vi "Main.vi"() -> ()   [LabVIEW 2020]
doc: "Ce VI modèle est conçu pour le modèle de conception Gestionnaire de messages dans une file d'attente.\n\nLa boucle de gestion d'événements génère des messages en fonction des actions sur l'interface utilisateur.\n\nLa boucle de gestion de messages traite les messages générés par la boucle de gestion d'événements ou par d'autres messages. Les messages sont des valeurs chaîne ; il est donc facile d'ajouter de nouveaux messages à la structure condition Conditions de messages de la boucle de gestion de messages Chaque cluster Message peut en outre fournir une valeur optionnelle pour Données de message, un variant qui peut être converti aux données requises pour un message spécifique."
uses:
  controls/Ctrl_Display.ctl
  controls/Ctrl_RefPad.ctl
  <vilib>/Utility/error.llb/Error Cluster From Error Code.vi
  support/Message Queue/Enqueue Message (Single).vi
  <vilib>/ErrorRing/Error Ring.xnode
  support/Message Queue/Message Queue.lvlib
  support/User Event - Stop/User Event - Stop.lvlib
panel:
  out "sortie d'erreur 2":errorcluster caption="sortie d'erreur"
  in  "Btn_Error_etat":bool caption="Error state"
  in  "Btn_Error":bool caption="Error"
  out "sortie d'erreur":errorcluster
  out "Display":T1
  in  "Pad":T2
  in  "Btn_Stop":bool
  # "Calculatrice"
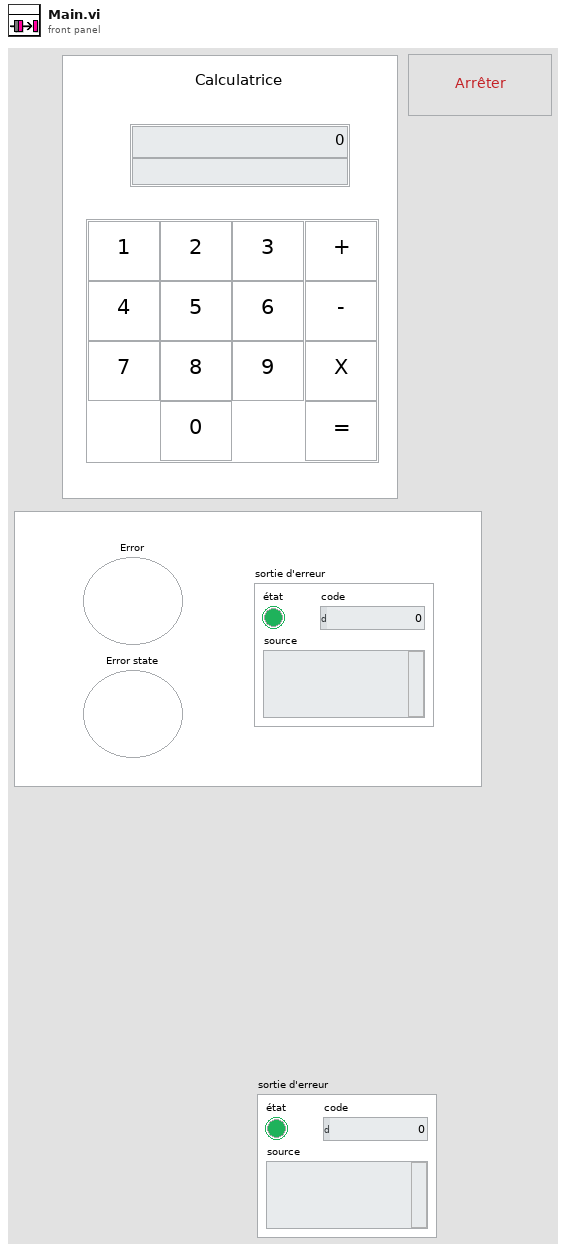
[diagram p1: front panel]
types:
  T1 = typedef "Ctrl_Display.ctl" = cluster{"Num":dbl, "Char":string}
  T2 = cluster{"Btn_1":bool, "Btn_2":bool, "Btn_3":bool, "Btn_4":bool, "Btn_5":bool, "Btn_6":bool, "Btn_7":bool, "Btn_8":bool, "Btn_9":bool, "Btn_0":bool, "Btn_+":bool, "Btn_-":bool, "Btn_X":bool, "Btn_=":bool}
  T3 = cluster{"état":bool, "code":i32, "source":string}
  T4 = typedef "Message Queue.lvlib/All Message Queues.ctl" = cluster{"Conductor":refnum<queue>, "IU":refnum<queue>}
  T5 = typedef "Ctrl_RefPad.ctl" = cluster{"BTN_Ref":refnum<vi>, "CharPad":string}
  T6 = typedef "UI Data.ctl" = cluster{"Data":cluster{"memory":string, "Display":T1}, "Ref":T7}
  T7 = typedef "Ctrl_Ref.ctl" = cluster{"Fifo":T4, "Event":cluster{"Stop":refnum<user-event>}}
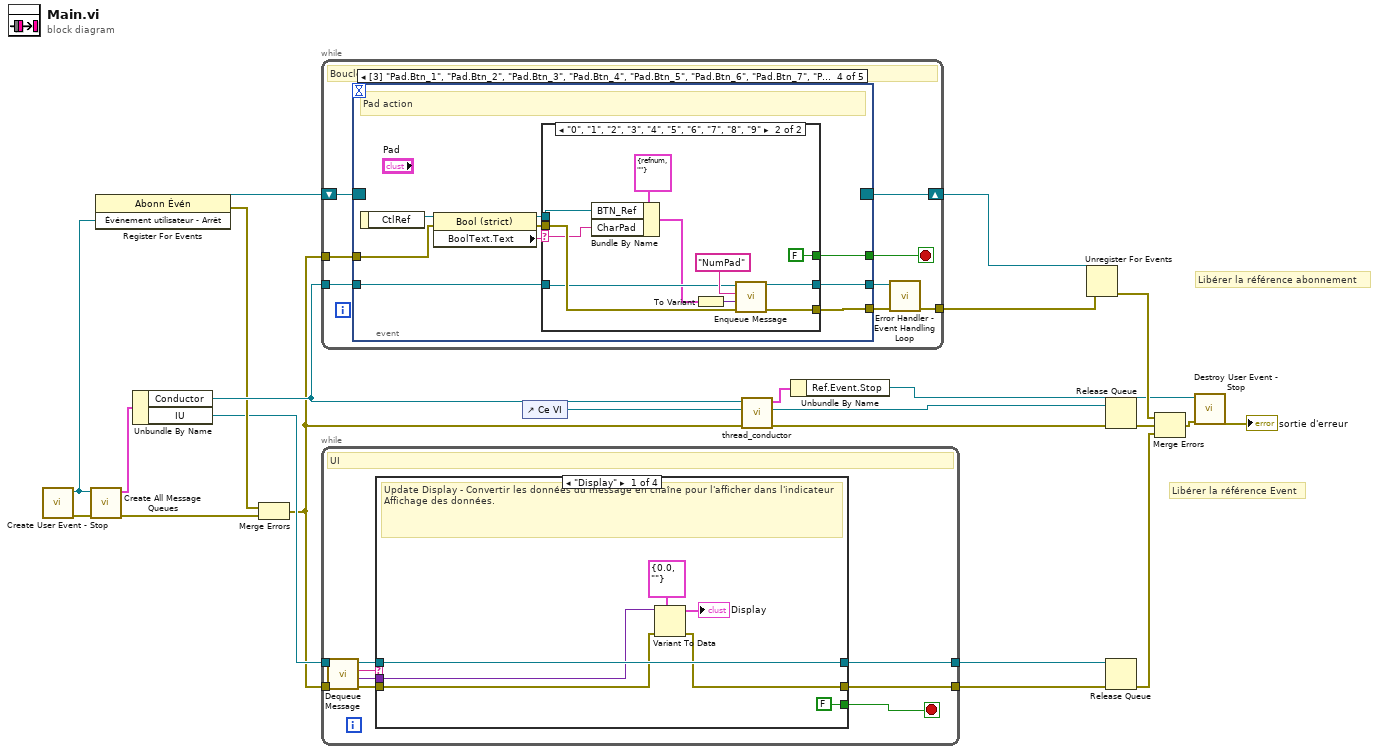
[diagram p0: block diagram]
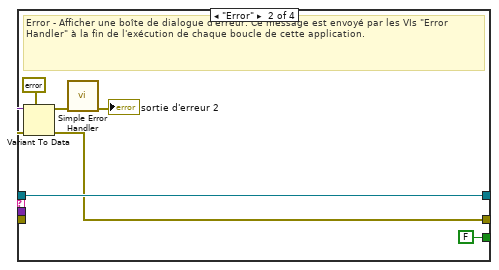
[diagram p2: hidden frame]
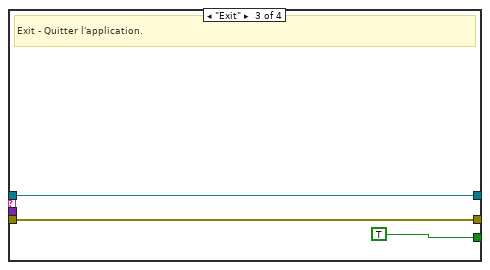
[diagram p3: hidden frame]
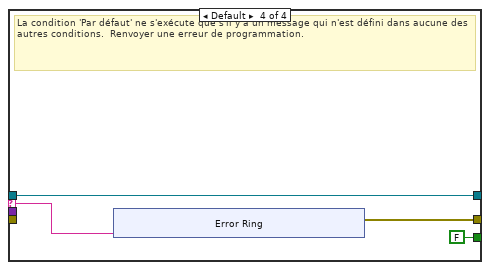
[diagram p4: hidden frame]
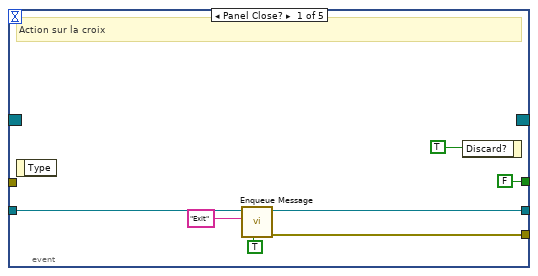
[diagram p5: hidden frame]
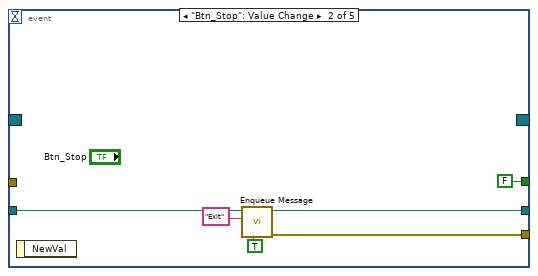
[diagram p6: hidden frame]
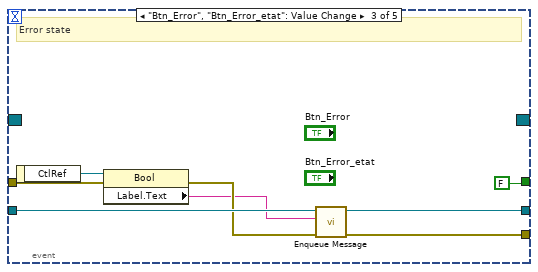
[diagram p7: hidden frame]
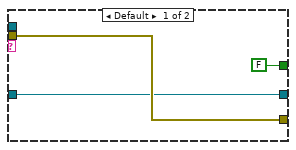
[diagram p8: hidden frame]
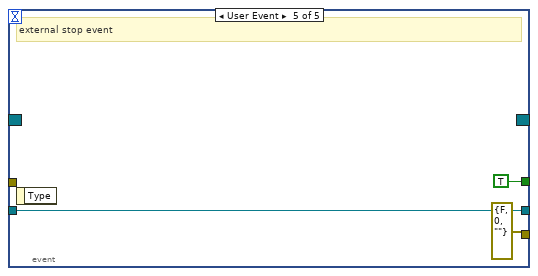
[diagram p9: hidden frame]
diagram:
  # "Libérer la référence abonnement"
  # "Libérer la référence Event"
  n1 = call "Create User Event - Stop.vi"() -> ("error out"=w20:T3, "Événement utilisateur - Arrêt"=w13:refnum<user-event>)  [unwired: 10 in]
  n2 = call "Create All Message Queues.vi"("error in (no error)"=w20, "Stop Event"=w13) -> ("error out"=w23:T3, "Fifo"=w22:T4)  [unwired: 8 in]
  n3 = register-events(w13) -> (reference out=w15:refnum<event-registration>, error out=w14:errorcluster)  [unwired: 2 in]
  n4 = Unbundle By Name(w22) -> ("Conductor"=w21:refnum<queue>, "IU"=w9:refnum<queue>)
  n5 = Merge Errors(w14, w23) -> (w8:errorcluster)
  n6 = while {
    tunnel: w21 -> [w31]
    shift-right: [w29] -> w17
    shift-left: w15 -> [w30]
    tunnel: [w25] -> w16
    tunnel: w8 -> [w24]
    stop <- w27 stop-if-true
    # "Boucle de gestion d'événements"
    n7 = event shown="[3] \"Pad.Btn_1\", \"Pad.Btn_2\", \"Pad.Btn_3\", \"Pad.Btn_4\", \"Pad.Btn_5\", \"Pad.Btn_6\", \"Pad.Btn_7\", \"Pad.Btn_8\", \"Pad.Btn_9\", \"Pad.Btn_0\", \"Pad.Btn_+\": Valeur changée" {
      selector: w30 -> [_ _ _ _ _]
      dyn-events: [_ _ _ _ _] -> w29
      timeout: _ -> [_ _ _ _ _]
      tunnel: [FALSE ("Discard?") FALSE ("Discard?") FALSE w54 TRUE ("Discard?")] -> w27
      tunnel: w31 -> [w37 w44 w50 w56 w78]
      tunnel: [w36 w43 w45 w57 T3 {"état"=FALSE, "code"=0, "source"=""} ("error out")] -> w28
      tunnel: [w35 w42 w49 w55 w78] -> w26
      tunnel: w24 -> [_ _ w51 w60 _]
      event Panel Close? {
        # "Action sur la croix"
        n8 = event-data() -> ()  [unwired: 1 in, 1 out]
        n9 = call-poly "Enqueue Message.vi"("Message prioritaire ? (F)"=TRUE ("Priority Message? (F)"), "Message"="Exit", "File d'attente de messages"=w37) -> ("error out"=w36:T3, "File d'attente de message dup."=w35:refnum<queue>)  [unwired: 7 in]
        n10 = event-data ("Event Filter Node")("Discard?"=TRUE) -> ()  [unwired: 1 in, 1 out]
      }
      event "Btn_Stop": Value Change {
        n11 = event-data() -> ()  [unwired: 1 in, 1 out]
        n12 = call-poly "Enqueue Message.vi"("Message prioritaire ? (F)"=TRUE ("Priority Message? (F)"), "Message"="Exit", "File d'attente de messages"=w44) -> ("error out"=w43:T3, "File d'attente de message dup."=w42:refnum<queue>)  [unwired: 7 in]
      }
      event "Btn_Error", "Btn_Error_etat": Value Change {
        # "Error state"
        n13 = event-data() -> ("CtlRef"=w52:refnum<vi>)  [unwired: 1 in]
        n14 = property class="Bool"(reference=w52, error in=w51) -> (error out=w48:errorcluster, "Label.Text"=w47:string)  [unwired: 1 out]
        n15 = call-poly "Enqueue Message.vi"("error in (no error)"=w48, "Message"=w47, "File d'attente de messages"=w50) -> ("error out"=w45:T3, "File d'attente de message dup."=w49:refnum<queue>)  [unwired: 7 in]
      }
      event "Pad.Btn_1", "Pad.Btn_2", "Pad.Btn_3", "Pad.Btn_4", "Pad.Btn_5", "Pad.Btn_6", "Pad.Btn_7", "Pad.Btn_8", "Pad.Btn_9", "Pad.Btn_0", "Pad.Btn_+": Value Change {
        # "Pad action"
        n16 = event-data() -> ("CtlRef"=w61:refnum<vi>)  [unwired: 1 in]
        n17 = property class="Bool (strict)"(reference=w61, error in=w60) -> (reference out=w53:refnum<vi>, error out=w58:errorcluster, "BoolText.Text"=w59:string)
        n18 = case shown="\"0\", \"1\", \"2\", \"3\", \"4\", \"5\", \"6\", \"7\", \"8\", \"9\"" w59 {
          selector: w59 -> [_ w67]
          tunnel: w58 -> [w64 w74]
          tunnel: [w64 w73] -> w57
          tunnel: w56 -> [w63 w71]
          tunnel: [w63 w70] -> w55
          tunnel: [FALSE FALSE] -> w54
          tunnel: w53 -> [_ w68]
          frame Default {
          }
          frame "0", "1", "2", "3", "4", "5", "6", "7", "8", "9" {
            n19 = Bundle By Name(cluster=T5 {"BTN_Ref"=refnum, "CharPad"=""}, "BTN_Ref"=w68, "CharPad"=w67) -> (w66:T5)
            n20 = To Variant(anything=w66) -> (Variant=w72:variant)
            n21 = call-poly "Enqueue Message.vi"("error in (no error)"=w74, "Données de message"=w72, "Message"="NumPad", "File d'attente de messages"=w71) -> ("error out"=w73:T3, "File d'attente de message dup."=w70:refnum<queue>)  [unwired: 6 in]
          }
        }
      }
      event User Event {
        # "external stop event"
        n22 = event-data() -> ()  [unwired: 1 in, 1 out]
      }
    }
    n23 = call "Error Handler - Event Handling Loop.vi"("error in (no error)"=w28, "File d'attente de messages"=w26) -> ("erreur en entrée dup."=w25:T3)  [unwired: 8 in, 1 out]
  }
  n24 = while {
    tunnel: w9 -> [w85]
    tunnel: w8 -> [w86]
    tunnel: [w79] -> w6
    tunnel: [w80] -> w7
    stop <- w87 stop-if-true
    # "UI"
    n25 = call "Dequeue Message.vi"("error in (no error)"=w86, "File d'attente de messages"=w85) -> ("error out"=w84:T3, "Données de message"=w82:variant, "Message"=w83:string, "File d'attente de message dup."=w81:refnum<queue>)  [unwired: 6 in]
    n26 = case "Conditions des messages" shown="\"Display\"" w83 {
      selector: w83 -> [_ _ _ w108]
      tunnel: w81 -> [w93 w96 w104 w106]
      tunnel: w84 -> [w92 w102 w103 _]
      tunnel: [w91 w95 w103 w109] -> w79
      tunnel: [FALSE FALSE TRUE FALSE] -> w87
      tunnel: w82 -> [w90 w101 _ _]
      tunnel: [w93 w96 w104 w106] -> w80
      frame "Display" {
        # "Update Display - Convertir les données du message en chaîne pour l'afficher dans l'indicateur Affichage des données."
        n27 = Variant To Data(error in=w92, type=T1 {"Num"=0.0, "Char"=""} ("Display"), Variant=w90) -> (data=→"Display":T1, error out=w91:errorcluster)
      }
      frame "Error" {
        # "Error - Afficher une boîte de dialogue d'erreur. Ce message est envoyé par les VIs \"Error Handler\" à la fin de l'exécution de chaque boucle de cette application."
        n28 = Variant To Data(error in=w102, type=errorcluster {"status"=FALSE, "code"=0, "source"=""} ("error constant"), Variant=w101) -> (data=w99:errorcluster, error out=w95:errorcluster)
        n29 = call <vilib>:"Simple Error Handler.vi"("error in (no error)"=w99) -> ("error out"=→"sortie d'erreur 2":errorcluster)  [unwired: 4 in, 4 out]
      }
      frame "Exit" {
        # "Exit - Quitter l'application."
      }
      frame Default {
        # "La condition 'Par défaut' ne s'exécute que s'il y a un message qui n'est défini dans aucune des autres conditions.  Renvoyer une erreur de programmation."
        n30 = xnode ("Error Ring")("paramètre 0"=w108) -> ("sortie d'erreur"=w109:errorcluster)
      }
    }
  }
  n31 = control-ref of="Ce VI"() -> (w3:refnum<vi>)
  n32 = call "thread_conductor.vi"("entrée d'erreur (pas d'erreur)"=w8, "Ce VI"=w3, "File d'attente en entrée"=w21) -> ("sortie d'erreur"=w11:T3, "File d'attente en sortie"=w1:refnum<queue>, "Data Cluster"=w2:T6)  [unwired: 6 in]
  n33 = Unbundle By Name(w2) -> ("Ref.Event.Stop"=w12:refnum<user-event>)
  n34 = Unregister For Events(event registration refnum=w17, error in=w16) -> (error out=w18:errorcluster)
  n35 = Release Queue(queue=w1, error in (no error)=w11) -> (error out=w10:errorcluster)  [unwired: 1 in, 2 out]
  n36 = Release Queue(queue=w7, error in (no error)=w6) -> (error out=w5:errorcluster)  [unwired: 1 in, 2 out]
  n37 = Merge Errors(w18, w10, w5) -> (w19:errorcluster)
  n38 = call "Destroy User Event - Stop.vi"("error in (no error)"=w19, "Événement utilisateur - Arrêt"=w12) -> ("error out"=→"sortie d'erreur":T3)  [unwired: 9 in]
